vi "PathPlanner_Cmd_FollowHolonomicPathExecute.vi"(5 "PathPlanner_Cmd_FollowHolConfig":T22={"HOLONOMIC_CTRL_PACK_TUNING"={"X PID Tuning"={"Kp"=0.0, "Ki"=0.0, "Kd"=0.0, "MaximumIntegral"=9.9e+30, "MinimumIntegral"=-9.9e+30, "IntegralZone"=9.9e+30}, "Y PID Tuning"={"Kp"=0.0, "Ki"=0.0, "Kd"=0.0, "MaximumIntegral"=9.9e+30, "MinimumIntegral"=-9.9e+30, "IntegralZone"=9.9e+30}, "thetaProfiledPID_CTRL"={"Controller"={"Kp"=0.0, "Ki"=0.0, "Kd"=0.0, "Period"=0.0, "Max_Integral"=1.0, "Min_Integral"=-1.0, "Max_Input"=0.0, "Min_Input"=0.0, "Continuous"=FALSE, "PositionError"=0.0, "VelocityError"=0.0, "PrevError"=0.0, "Total_Integral"=0.0, "PositionTolerance"=0.05, "VelocityTolerance"=9.99e+35, "SetPoint"=0.0, "Kf"=0.0, "Prev_Deriv"=0.0, "Prev_Deriv 2"=0.0, "DerivativeFilter"=FALSE, "Min_Output"=-9.99e+35, "Max_Output"=9.9e+35, "Prev_F_P"=0.0, "Prev_F_P_2"=0.0, "AntiWindupActive"=FALSE, "Measurement"=0.0, "IntegralZone"=9.9e+30}, "Goal"={"Position"=0.0, "Velocity"=0.0}, "Setpoint"={"Position"=0.0, "Velocity"=0.0}, "Constraint"={"MaxVelocity"=0.0, "MaxAcceleration"=0.0}}}, "Max Wheel Speed M/S"=0.0, "Tolerance SI"={"TRANSLATION"={"X"=0.04, "Y"=0.04}, "ROTATION"={"VALUE"=0.034906585039887, "COS"=0.999390827019096, "SIN"=0.034899496702501}}, "Drive Base Radius M"=0.0, "ControlPastEnd_Sec"=3.0, "ReplanningConfig"={"enableInitialReplanning"=FALSE, "enableDynamicReplanning"=FALSE, "dynamicReplanningTotalErrorThreshold"=0.0, "dynamicReplanningErrorSpikeThreshold"=0.0}, "Period_Sec"=0.02, "Trigger Events"=TRUE} {"Tolerance SI"."ROTATION"."SIN" format="%13.4f"; "Tolerance SI"."ROTATION"."COS" format="%13.4f"; "Tolerance SI"."ROTATION"."VALUE" format="%13.4f"; "Tolerance SI"."TRANSLATION"."Y" format="%14.3f"; "Tolerance SI"."TRANSLATION"."X" format="%14.3f"; "HOLONOMIC_CTRL_PACK_TUNING"."thetaProfiledPID_CTRL"."Constraint"."MaxAcceleration" format="%16_6e"; "HOLONOMIC_CTRL_PACK_TUNING"."thetaProfiledPID_CTRL"."Constraint"."MaxVelocity" format="%16_6e"; "HOLONOMIC_CTRL_PACK_TUNING"."thetaProfiledPID_CTRL"."Setpoint"."Velocity" format="%16_6e"; "HOLONOMIC_CTRL_PACK_TUNING"."thetaProfiledPID_CTRL"."Setpoint"."Position" format="%16_6e"; "HOLONOMIC_CTRL_PACK_TUNING"."thetaProfiledPID_CTRL"."Goal"."Velocity" format="%16_6e"; "HOLONOMIC_CTRL_PACK_TUNING"."thetaProfiledPID_CTRL"."Goal"."Position" format="%16_6e"; "HOLONOMIC_CTRL_PACK_TUNING"."thetaProfiledPID_CTRL"."Controller"."IntegralZone" format="%16_6e"; "HOLONOMIC_CTRL_PACK_TUNING"."thetaProfiledPID_CTRL"."Controller"."Measurement" format="%16_6e"; "HOLONOMIC_CTRL_PACK_TUNING"."thetaProfiledPID_CTRL"."Controller"."Prev_F_P_2" format="%16_6e"; "HOLONOMIC_CTRL_PACK_TUNING"."thetaProfiledPID_CTRL"."Controller"."Prev_F_P" format="%16_6e"; "HOLONOMIC_CTRL_PACK_TUNING"."thetaProfiledPID_CTRL"."Controller"."Max_Output" format="%16_6e"; "HOLONOMIC_CTRL_PACK_TUNING"."thetaProfiledPID_CTRL"."Controller"."Min_Output" format="%16_6e"; "HOLONOMIC_CTRL_PACK_TUNING"."thetaProfiledPID_CTRL"."Controller"."Prev_Deriv 2" format="%16_6e"; "HOLONOMIC_CTRL_PACK_TUNING"."thetaProfiledPID_CTRL"."Controller"."Prev_Deriv" format="%16_6e"; "HOLONOMIC_CTRL_PACK_TUNING"."thetaProfiledPID_CTRL"."Controller"."Kf" format="%16_6e"; "HOLONOMIC_CTRL_PACK_TUNING"."thetaProfiledPID_CTRL"."Controller"."SetPoint" format="%16_6e"; "HOLONOMIC_CTRL_PACK_TUNING"."thetaProfiledPID_CTRL"."Controller"."VelocityTolerance" format="%16_6e"; "HOLONOMIC_CTRL_PACK_TUNING"."thetaProfiledPID_CTRL"."Controller"."PositionTolerance" format="%16_6e"; "HOLONOMIC_CTRL_PACK_TUNING"."thetaProfiledPID_CTRL"."Controller"."Total_Integral" format="%16_6e"; "HOLONOMIC_CTRL_PACK_TUNING"."thetaProfiledPID_CTRL"."Controller"."PrevError" format="%16_6e"; "HOLONOMIC_CTRL_PACK_TUNING"."thetaProfiledPID_CTRL"."Controller"."VelocityError" format="%16_6e"; "HOLONOMIC_CTRL_PACK_TUNING"."thetaProfiledPID_CTRL"."Controller"."PositionError" format="%16_6e"; "HOLONOMIC_CTRL_PACK_TUNING"."thetaProfiledPID_CTRL"."Controller"."Min_Input" format="%16_6e"; "HOLONOMIC_CTRL_PACK_TUNING"."thetaProfiledPID_CTRL"."Controller"."Max_Input" format="%16_6e"; "HOLONOMIC_CTRL_PACK_TUNING"."thetaProfiledPID_CTRL"."Controller"."Min_Integral" format="%16_6e"; "HOLONOMIC_CTRL_PACK_TUNING"."thetaProfiledPID_CTRL"."Controller"."Max_Integral" format="%16_6e"; "HOLONOMIC_CTRL_PACK_TUNING"."thetaProfiledPID_CTRL"."Controller"."Period" format="%16_6e"; "HOLONOMIC_CTRL_PACK_TUNING"."thetaProfiledPID_CTRL"."Controller"."Kd" format="%16_6e"; "HOLONOMIC_CTRL_PACK_TUNING"."thetaProfiledPID_CTRL"."Controller"."Ki" format="%16_6e"; "HOLONOMIC_CTRL_PACK_TUNING"."thetaProfiledPID_CTRL"."Controller"."Kp" format="%16_6e"}, 6 "PassthroughTime_SEC":dbl=-1.0, 7 "PathPlannerPath":T2={"Reversed"=FALSE, "RotationTargets"=[], "ConstraintZones"=[], "EventMarkers"=[], "GlobalConstraints"={"MaxVelocityMps;"=0.0, "MaxAccelerationMpsSq;"=0.0, "MaxAngularVelRadPsEc;"=0.0, "MaxAngularAccRadPSecSq"=0.0, "Exists"=FALSE, "Unlimited"=FALSE, "NominalVoltageVolts"=12.0}, "GoalEndState"={"VelocityMPS"=0.0, "Rotation"={"VALUE"=0.0, "COS"=1.0, "SIN"=0.0}}, "AllPoints"=[], "Name"="", "Waypoints"=[], "PointTowardsZones"=[], "IdealStartingState"={"VelocityMPS"=0.0, "Rotation"={"VALUE"=1.0, "COS"=0.0, "SIN"=0.0}}, "IsChoreoPath"=FALSE, "PreventFlipping"=FALSE} {"IdealStartingState"."Rotation"."SIN" format="%13.4f"; "IdealStartingState"."Rotation"."COS" format="%13.4f"; "IdealStartingState"."Rotation"."VALUE" format="%13.4f"; "PointTowardsZones"."TargetPosition"."Y" format="%14.3f"; "PointTowardsZones"."TargetPosition"."X" format="%14.3f"; "PointTowardsZones"."RotationOffset"."SIN" format="%13.4f"; "PointTowardsZones"."RotationOffset"."COS" format="%13.4f"; "PointTowardsZones"."RotationOffset"."VALUE" format="%13.4f"; "Waypoints"."nextControl"."Y" format="%14.3f"; "Waypoints"."nextControl"."X" format="%14.3f"; "Waypoints"."anchor"."Y" format="%14.3f"; "Waypoints"."anchor"."X" format="%14.3f"; "Waypoints"."prevControl"."Y" format="%14.3f"; "Waypoints"."prevControl"."X" format="%14.3f"; "AllPoints"."RotationTarget"."rotation"."SIN" format="%13.4f"; "AllPoints"."RotationTarget"."rotation"."COS" format="%13.4f"; "AllPoints"."RotationTarget"."rotation"."VALUE" format="%13.4f"; "AllPoints"."Position"."Y" format="%14.3f"; "AllPoints"."Position"."X" format="%14.3f"; "GoalEndState"."Rotation"."SIN" format="%13.4f"; "GoalEndState"."Rotation"."COS" format="%13.4f"; "GoalEndState"."Rotation"."VALUE" format="%13.4f"; "RotationTargets"."rotation"."SIN" format="%13.4f"; "RotationTargets"."rotation"."COS" format="%13.4f"; "RotationTargets"."rotation"."VALUE" format="%13.4f"}, 8 "Enabled":bool=TRUE, 9 "Reset":bool, 10 "CurrentChassisSpeeds":T1 {"vOmega" format="%10.3f"; "vY" format="%10.3f"; "vX" format="%10.3f"}, 11 "Current Pose SI":T17={"TRANSLATION"={"X"=0.0, "Y"=0.0}, "ROTATION"={"VALUE"=0.0, "COS"=1.0, "SIN"=0.0}} {"ROTATION"."SIN" format="%13.4f"; "ROTATION"."COS" format="%13.4f"; "ROTATION"."VALUE" format="%13.4f"; "TRANSLATION"."Y" format="%14.3f"; "TRANSLATION"."X" format="%14.3f"}) -> (0 "Position Error M":dbl, 1 "Complete":bool, 2 "At Reference":bool, 3 "calcChassisSpeed":T1 {"vOmega" format="%10.3f"; "vY" format="%10.3f"; "vX" format="%10.3f"}, 4 "outHOLONOMIC_DRV_CTRL":T16={"poseTolerance"={"TRANSLATION"={"X"=0.0, "Y"=0.0}, "ROTATION"={"VALUE"=0.0, "COS"=1.0, "SIN"=0.0}}, "poseError"={"TRANSLATION"={"X"=0.0, "Y"=0.0}, "ROTATION"={"VALUE"=0.0, "COS"=1.0, "SIN"=0.0}}, "Enabled"=TRUE, "PID_xCtrl"={"Kp"=0.0, "Ki"=0.0, "Kd"=0.0, "Period"=0.0, "Max_Integral"=1.0, "Min_Integral"=-1.0, "Max_Input"=0.0, "Min_Input"=0.0, "Continuous"=FALSE, "PositionError"=0.0, "VelocityError"=0.0, "PrevError"=0.0, "Total_Integral"=0.0, "PositionTolerance"=0.05, "VelocityTolerance"=9.99e+35, "SetPoint"=0.0, "Kf"=0.0, "Prev_Deriv"=0.0, "Prev_Deriv 2"=0.0, "DerivativeFilter"=FALSE, "Min_Output"=-9.99e+35, "Max_Output"=9.9e+35, "Prev_F_P"=0.0, "Prev_F_P_2"=0.0, "AntiWindupActive"=FALSE, "Measurement"=0.0, "IntegralZone"=9.9e+30}, "PID_yCtrl"={"Kp"=0.0, "Ki"=0.0, "Kd"=0.0, "Period"=0.0, "Max_Integral"=1.0, "Min_Integral"=-1.0, "Max_Input"=0.0, "Min_Input"=0.0, "Continuous"=FALSE, "PositionError"=0.0, "VelocityError"=0.0, "PrevError"=0.0, "Total_Integral"=0.0, "PositionTolerance"=0.05, "VelocityTolerance"=9.99e+35, "SetPoint"=0.0, "Kf"=0.0, "Prev_Deriv"=0.0, "Prev_Deriv 2"=0.0, "DerivativeFilter"=FALSE, "Min_Output"=-9.99e+35, "Max_Output"=9.9e+35, "Prev_F_P"=0.0, "Prev_F_P_2"=0.0, "AntiWindupActive"=FALSE, "Measurement"=0.0, "IntegralZone"=9.9e+30}, "PROF_PID_thetaCtrl"={"Controller"={"Kp"=0.0, "Ki"=0.0, "Kd"=0.0, "Period"=0.0, "Max_Integral"=1.0, "Min_Integral"=-1.0, "Max_Input"=0.0, "Min_Input"=0.0, "Continuous"=FALSE, "PositionError"=0.0, "VelocityError"=0.0, "PrevError"=0.0, "Total_Integral"=0.0, "PositionTolerance"=0.05, "VelocityTolerance"=9.99e+35, "SetPoint"=0.0, "Kf"=0.0, "Prev_Deriv"=0.0, "Prev_Deriv 2"=0.0, "DerivativeFilter"=FALSE, "Min_Output"=-9.99e+35, "Max_Output"=9.9e+35, "Prev_F_P"=0.0, "Prev_F_P_2"=0.0, "AntiWindupActive"=FALSE, "Measurement"=0.0, "IntegralZone"=9.9e+30}, "Goal"={"Position"=0.0, "Velocity"=0.0}, "Setpoint"={"Position"=0.0, "Velocity"=0.0}, "Constraint"={"MaxVelocity"=0.0, "MaxAcceleration"=0.0}}, "RotationError"={"VALUE"=0.0, "COS"=1.0, "SIN"=0.0}, "FirstRun"=TRUE} {"RotationError"."SIN" format="%13.4f"; "RotationError"."COS" format="%13.4f"; "RotationError"."VALUE" format="%13.4f"; "PROF_PID_thetaCtrl"."Constraint"."MaxAcceleration" format="%16_6e"; "PROF_PID_thetaCtrl"."Constraint"."MaxVelocity" format="%16_6e"; "PROF_PID_thetaCtrl"."Setpoint"."Velocity" format="%16_6e"; "PROF_PID_thetaCtrl"."Setpoint"."Position" format="%16_6e"; "PROF_PID_thetaCtrl"."Goal"."Velocity" format="%16_6e"; "PROF_PID_thetaCtrl"."Goal"."Position" format="%16_6e"; "PROF_PID_thetaCtrl"."Controller"."IntegralZone" format="%16_6e"; "PROF_PID_thetaCtrl"."Controller"."Measurement" format="%16_6e"; "PROF_PID_thetaCtrl"."Controller"."Prev_F_P_2" format="%16_6e"; "PROF_PID_thetaCtrl"."Controller"."Prev_F_P" format="%16_6e"; "PROF_PID_thetaCtrl"."Controller"."Max_Output" format="%16_6e"; "PROF_PID_thetaCtrl"."Controller"."Min_Output" format="%16_6e"; "PROF_PID_thetaCtrl"."Controller"."Prev_Deriv 2" format="%16_6e"; "PROF_PID_thetaCtrl"."Controller"."Prev_Deriv" format="%16_6e"; "PROF_PID_thetaCtrl"."Controller"."Kf" format="%16_6e"; "PROF_PID_thetaCtrl"."Controller"."SetPoint" format="%16_6e"; "PROF_PID_thetaCtrl"."Controller"."VelocityTolerance" format="%16_6e"; "PROF_PID_thetaCtrl"."Controller"."PositionTolerance" format="%16_6e"; "PROF_PID_thetaCtrl"."Controller"."Total_Integral" format="%16_6e"; "PROF_PID_thetaCtrl"."Controller"."PrevError" format="%16_6e"; "PROF_PID_thetaCtrl"."Controller"."VelocityError" format="%16_6e"; "PROF_PID_thetaCtrl"."Controller"."PositionError" format="%16_6e"; "PROF_PID_thetaCtrl"."Controller"."Min_Input" format="%16_6e"; "PROF_PID_thetaCtrl"."Controller"."Max_Input" format="%16_6e"; "PROF_PID_thetaCtrl"."Controller"."Min_Integral" format="%16_6e"; "PROF_PID_thetaCtrl"."Controller"."Max_Integral" format="%16_6e"; "PROF_PID_thetaCtrl"."Controller"."Period" format="%16_6e"; "PROF_PID_thetaCtrl"."Controller"."Kd" format="%16_6e"; "PROF_PID_thetaCtrl"."Controller"."Ki" format="%16_6e"; "PROF_PID_thetaCtrl"."Controller"."Kp" format="%16_6e"; "PID_yCtrl"."IntegralZone" format="%16_6e"; "PID_yCtrl"."Measurement" format="%16_6e"; "PID_yCtrl"."Prev_F_P_2" format="%16_6e"; "PID_yCtrl"."Prev_F_P" format="%16_6e"; "PID_yCtrl"."Max_Output" format="%16_6e"; "PID_yCtrl"."Min_Output" format="%16_6e"; "PID_yCtrl"."Prev_Deriv 2" format="%16_6e"; "PID_yCtrl"."Prev_Deriv" format="%16_6e"; "PID_yCtrl"."Kf" format="%16_6e"; "PID_yCtrl"."SetPoint" format="%16_6e"; "PID_yCtrl"."VelocityTolerance" format="%16_6e"; "PID_yCtrl"."PositionTolerance" format="%16_6e"; "PID_yCtrl"."Total_Integral" format="%16_6e"; "PID_yCtrl"."PrevError" format="%16_6e"; "PID_yCtrl"."VelocityError" format="%16_6e"; "PID_yCtrl"."PositionError" format="%16_6e"; "PID_yCtrl"."Min_Input" format="%16_6e"; "PID_yCtrl"."Max_Input" format="%16_6e"; "PID_yCtrl"."Min_Integral" format="%16_6e"; "PID_yCtrl"."Max_Integral" format="%16_6e"; "PID_yCtrl"."Period" format="%16_6e"; "PID_yCtrl"."Kd" format="%16_6e"; "PID_yCtrl"."Ki" format="%16_6e"; "PID_yCtrl"."Kp" format="%16_6e"; "PID_xCtrl"."IntegralZone" format="%16_6e"; "PID_xCtrl"."Measurement" format="%16_6e"; "PID_xCtrl"."Prev_F_P_2" format="%16_6e"; "PID_xCtrl"."Prev_F_P" format="%16_6e"; "PID_xCtrl"."Max_Output" format="%16_6e"; "PID_xCtrl"."Min_Output" format="%16_6e"; "PID_xCtrl"."Prev_Deriv 2" format="%16_6e"; "PID_xCtrl"."Prev_Deriv" format="%16_6e"; "PID_xCtrl"."Kf" format="%16_6e"; "PID_xCtrl"."SetPoint" format="%16_6e"; "PID_xCtrl"."VelocityTolerance" format="%16_6e"; "PID_xCtrl"."PositionTolerance" format="%16_6e"; "PID_xCtrl"."Total_Integral" format="%16_6e"; "PID_xCtrl"."PrevError" format="%16_6e"; "PID_xCtrl"."VelocityError" format="%16_6e"; "PID_xCtrl"."PositionError" format="%16_6e"; "PID_xCtrl"."Min_Input" format="%16_6e"; "PID_xCtrl"."Max_Input" format="%16_6e"; "PID_xCtrl"."Min_Integral" format="%16_6e"; "PID_xCtrl"."Max_Integral" format="%16_6e"; "PID_xCtrl"."Period" format="%16_6e"; "PID_xCtrl"."Kd" format="%16_6e"; "PID_xCtrl"."Ki" format="%16_6e"; "PID_xCtrl"."Kp" format="%16_6e"; "poseError"."ROTATION"."SIN" format="%13.4f"; "poseError"."ROTATION"."COS" format="%13.4f"; "poseError"."ROTATION"."VALUE" format="%13.4f"; "poseError"."TRANSLATION"."Y" format="%14.3f"; "poseError"."TRANSLATION"."X" format="%14.3f"; "poseTolerance"."ROTATION"."SIN" format="%13.4f"; "poseTolerance"."ROTATION"."COS" format="%13.4f"; "poseTolerance"."ROTATION"."VALUE" format="%13.4f"; "poseTolerance"."TRANSLATION"."Y" format="%14.3f"; "poseTolerance"."TRANSLATION"."X" format="%14.3f"})   [LabVIEW 2019, in "PathPlanner24.lvlib"]
doc: "DOCUMENTATION IS NOT COMPLETE.\n \nCalculates the next output of the path following controller for holonomic drive robots. This wraps a Holonomic Drive Control function with the particulars needed to follow a PathPlanner trajectory.\n\nInputs:\n - PathPlanner_Holonomic_Ctrl_Pack_Tuning - cluster - The tuning paraameters for the holonomic drive controller. These are static. They should not be changed after the first call to this function.\n - CurrentPoseSi - pose2d - The current pose calculated by odometry or pose estimation. The pose can be absolute or relative depending on what type of trajectory is being followed.\n - PathPlannerState - cluster - The path palnner trajectory state containing the desired position and velocities of the robot.\n - Reset - boolean - When TRUE the holonomic drive controller is reset. This should be set to TRUE for the first execution of a trajectory.\n - Enabled - boolean - When TRUE, closed loop control is enabled. (Optional. Default: TRUE)\n - Period - double - The loop period in seconds for this controller. (Optional. Default: 0.020)\n\nOutputs:\n - CalcChassisSpeed - cluster - The desired chassis speed in SI units.\n - AtReference - boolean - TRUE if the robots position is within the defined tolerance.\n - PositionError - pose2d - Position error in SI units. How far the robot is away from the desired trajectory position.\n - out_Holonomic_Drive_Ctrl - THe current holonomic drive controller data cluster. This is mainly for diagnostic purposes."
uses:
  PathPlanner24.lvlib
  <vilib>/Rock Robotics/WPI/ThirdParty/JAS_Junk/TrajLib/TypeDef/TRANSLATION2D.ctl
  <vilib>/Rock Robotics/WPI/ThirdParty/JAS_Junk/TrajLib/Trajectory_Library.lvlib
  <vilib>/Rock Robotics/WPI/ThirdParty/JAS_Junk/TrajLib/TypeDef/ROTATION2D.ctl
  <vilib>/Rock Robotics/WPI/ThirdParty/JAS_Junk/TrajLib/TypeDef/POSE2D.ctl
  <vilib>/Rock Robotics/WPI/ThirdParty/JAS_Junk/TrajLib/TypeDef/PID_TUNING.ctl
  <vilib>/Rock Robotics/WPI/ThirdParty/JAS_Junk/TrajLib/TypeDef/PID_CONTROLLER.ctl
  <vilib>/Rock Robotics/WPI/ThirdParty/JAS_Junk/TrajLib/TypeDef/TRAPEZOID_PROFILE_STATE.ctl
  <vilib>/Rock Robotics/WPI/ThirdParty/JAS_Junk/TrajLib/TypeDef/TRAPEZOID_PROFILE_CONSTRAINT.ctl
  <vilib>/Rock Robotics/WPI/ThirdParty/JAS_Junk/TrajLib/TypeDef/PROFILED_PID_CONTROLLER.ctl
  <vilib>/Rock Robotics/WPI/ThirdParty/JAS_Junk/TrajLib/TypeDef/HOLONOMIC_PACK_TUNING.ctl
  <vilib>/Rock Robotics/WPI/ThirdParty/JAS_Junk/TrajLib/TypeDef/HOLONOMIC_DRV_CTRL.ctl
  <vilib>/Rock Robotics/WPI/ThirdParty/JAS_Junk/TrajLib/TypeDef/CHASSIS_SPEEDS.ctl
  TypeDef/PathPlannerRotationTarget.ctl
  TypeDef/PathPlannerPathConstraints.ctl
  TypeDef/PathPlannerConstraintsZone.ctl
  ENum/PathPlanner_CommandUtilType_ENUM.ctl
  TypeDef/PathPlannerCommandUtil.ctl
  TypeDef/PathPlannerEventMarker.ctl
  TypeDef/PathPlannerGoalEndState.ctl
  TypeDef/PathPlannerPathPoint.ctl
  TypeDef/PathPlannerPath.ctl
  TypeDef/PathPlannerCmdFollowHolConfig.ctl
  TypeDef/PathPlannerReplanningConfig.ctl
  TypeDef/PathPlannerWaypoint.ctl
  TypeDef/PathPlannerPointTowardsZone.ctl
  TypeDef/PathPlannerIdealStartingState.ctl
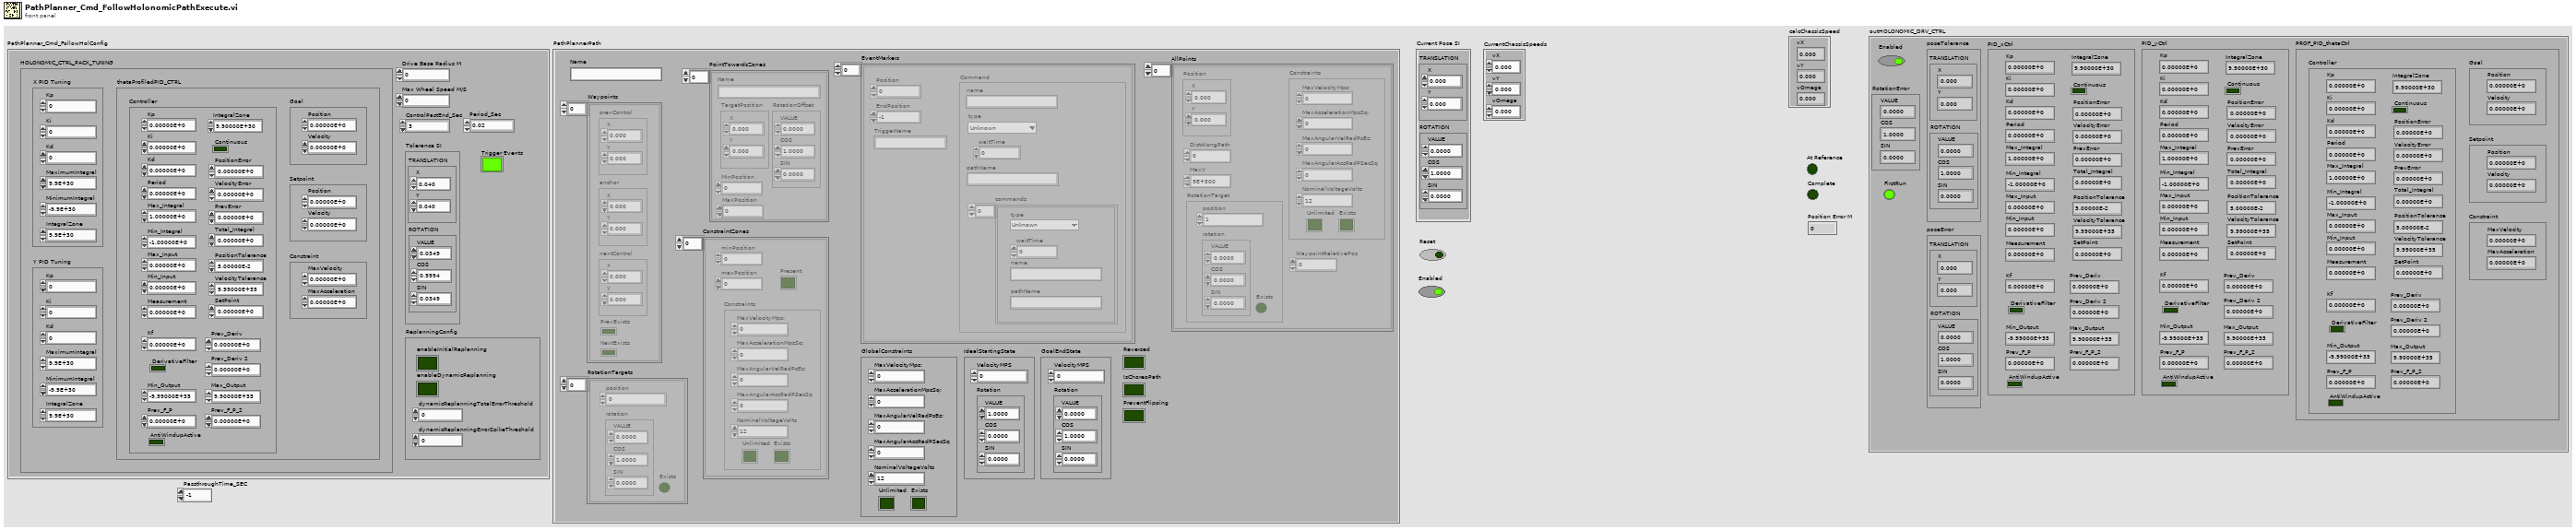
[diagram p1: front panel]
types:
  T1 = typedef "Trajectory_Library.lvlib/CHASSIS_SPEEDS.ctl" = cluster{"vX":dbl, "vY":dbl, "vOmega":dbl}
  T2 = typedef "PathPlanner24.lvlib/PathPlannerPath.ctl" = cluster{"Reversed":bool, "RotationTargets":T3[], "ConstraintZones":T5[], "EventMarkers":T7[], "GlobalConstraints":T6, "GoalEndState":T10, "AllPoints":T11[], "Name":string, "Waypoints":T13[], "PointTowardsZones":T14[], "IdealStartingState":T15, "IsChoreoPath":bool, "PreventFlipping":bool}
  T3 = typedef "PathPlanner24.lvlib/PathPlannerRotationTarget.ctl" = cluster{"position":dbl, "rotation":T4, "Exists":bool}
  T4 = typedef "Trajectory_Library.lvlib/ROTATION2D.ctl" = cluster{"VALUE":dbl, "COS":dbl, "SIN":dbl}
  T5 = typedef "PathPlanner24.lvlib/PathPlannerConstraintsZone.ctl" = cluster{"minPosition":dbl, "maxPosition":dbl, "Constraints":T6, "Present":bool}
  T6 = typedef "PathPlanner24.lvlib/PathPlannerPathConstraints.ctl" = cluster{"MaxVelocityMps;":dbl, "MaxAccelerationMpsSq;":dbl, "MaxAngularVelRadPsEc;":dbl, "MaxAngularAccRadPSecSq":dbl, "Exists":bool, "Unlimited":bool, "NominalVoltageVolts":dbl}
  T7 = typedef "PathPlanner24.lvlib/PathPlannerEventMarker.ctl" = cluster{"Position":dbl, "Command":T8, "TriggerName":string, "EndPosition":dbl}
  T8 = typedef "PathPlanner24.lvlib/PathPlannerCommandUtil.ctl" = cluster{"waitTime":dbl, "name":string, "pathName":string, "commands":cluster{"type":T9, "waitTime":dbl, "name":string, "pathName":string}[], "type":T9}
  T9 = typedef "PathPlanner24.lvlib/PathPlanner_CommandUtilType_ENUM.ctl" = enum16{"Unknown", "Wait", "Named", "Path", "Sequential", "Parallel", "Race", "Deadline"}
  T10 = typedef "PathPlanner24.lvlib/PathPlannerGoalEndState.ctl" = cluster{"VelocityMPS":dbl, "Rotation":T4}
  T11 = typedef "PathPlanner24.lvlib/PathPlannerPathPoint.ctl" = cluster{"Position":T12, "DistAlongPath":dbl, "MaxV":dbl, "Constraints":T6, "RotationTarget":T3, "WaypointRelativePos":dbl}
  T12 = typedef "Trajectory_Library.lvlib/TRANSLATION2D.ctl" = cluster{"X":dbl, "Y":dbl}
  T13 = typedef "PathPlanner24.lvlib/PathPlannerWaypoint.ctl" = cluster{"prevControl":T12, "anchor":T12, "nextControl":T12, "PrevExists":bool, "NextExists":bool}
  T14 = typedef "PathPlanner24.lvlib/PathPlannerPointTowardsZone.ctl" = cluster{"RotationOffset":T4, "Name":string, "TargetPosition":T12, "MinPosition":dbl, "MaxPosition":dbl}
  T15 = typedef "PathPlanner24.lvlib/PathPlannerIdealStartingState.ctl" = cluster{"VelocityMPS":dbl, "Rotation":T4}
  T16 = typedef "Trajectory_Library.lvlib/HOLONOMIC_DRV_CTRL.ctl" = cluster{"poseTolerance":T17, "poseError":T17, "Enabled":bool, "PID_xCtrl":T18, "PID_yCtrl":T18, "PROF_PID_thetaCtrl":T19, "RotationError":T4, "FirstRun":bool}
  T17 = typedef "Trajectory_Library.lvlib/POSE2D.ctl" = cluster{"TRANSLATION":T12, "ROTATION":T4}
  T18 = typedef "Trajectory_Library.lvlib/PID_CONTROLLER.ctl" = cluster{"Kp":dbl, "Ki":dbl, "Kd":dbl, "Period":dbl, "Max_Integral":dbl, "Min_Integral":dbl, "Max_Input":dbl, "Min_Input":dbl, "Continuous":bool, "PositionError":dbl, "VelocityError":dbl, "PrevError":dbl, "Total_Integral":dbl, "PositionTolerance":dbl, "VelocityTolerance":dbl, "SetPoint":dbl, "Kf":dbl, "Prev_Deriv":dbl, "Prev_Deriv 2":dbl, "DerivativeFilter":bool, "Min_Output":dbl, "Max_Output":dbl, "Prev_F_P":dbl, "Prev_F_P_2":dbl, "AntiWindupActive":bool, "Measurement":dbl, "IntegralZone":dbl}
  T19 = typedef "Trajectory_Library.lvlib/PROFILED_PID_CONTROLLER.ctl" = cluster{"Controller":T18, "Goal":T20, "Setpoint":T20, "Constraint":T21}
  T20 = typedef "Trajectory_Library.lvlib/TRAPEZOID_PROFILE_STATE.ctl" = cluster{"Position":dbl, "Velocity":dbl}
  T21 = typedef "Trajectory_Library.lvlib/TRAPEZOID_PROFILE_CONSTRAINT.ctl" = cluster{"MaxVelocity":dbl, "MaxAcceleration":dbl}
  T22 = typedef "PathPlanner24.lvlib/PathPlannerCmdFollowHolConfig.ctl" = cluster{"HOLONOMIC_CTRL_PACK_TUNING":T23, "Max Wheel Speed M/S":dbl, "Tolerance SI":T17, "Drive Base Radius M":dbl, "ControlPastEnd_Sec":dbl, "ReplanningConfig":T25, "Period_Sec":dbl, "Trigger Events":bool}
  T23 = typedef "Trajectory_Library.lvlib/HOLONOMIC_PACK_TUNING.ctl" = cluster{"X PID Tuning":T24, "Y PID Tuning":T24, "thetaProfiledPID_CTRL":T19}
  T24 = typedef "Trajectory_Library.lvlib/PID_TUNING.ctl" = cluster{"Kp":dbl, "Ki":dbl, "Kd":dbl, "MaximumIntegral":dbl, "MinimumIntegral":dbl, "IntegralZone":dbl}
  T25 = typedef "PathPlanner24.lvlib/PathPlannerReplanningConfig.ctl" = cluster{"enableInitialReplanning":bool, "enableDynamicReplanning":bool, "dynamicReplanningTotalErrorThreshold":dbl, "dynamicReplanningErrorSpikeThreshold":dbl}
  T26 = typedef "PathPlanner24.lvlib/PathPlannerCtrlHolConfig.ctl" = cluster{"HOLONOMIC_CTRL_PACK_TUNING":T23, "Max Wheel Speed M/S":dbl, "Tolerance SI":T17, "Drive Base Radius M":dbl}
  T27 = cluster{"Traj Time Plus Extra\nElapsed":bool, "Traj Time Elapsed":bool}
  T28 = typedef "PathPlanner24.lvlib/PathPlannerTrajectoryState24.ctl" = cluster{"TimeSeconds":dbl, "VelocityMPS":dbl, "AccerationMpsSq":dbl, "HeadingAngularVelRadPerSec":dbl, "PositionMeters":T12, "Heading":T4, "TargetHolonomicRotation":T4, "CurvatureRadPerMeter":dbl, "PathPlannerConstraints":T6, "DeltaPos":dbl}
  T29 = typedef "PathPlanner24.lvlib/PathPlannerTrajectoryEvents.ctl" = cluster{"EventCommands":T30[]}
  T30 = typedef "PathPlanner24.lvlib/PathPlannerTrajectoryEvent.ctl" = cluster{"TimeStampSec":dbl, "CommandUtil":T8}
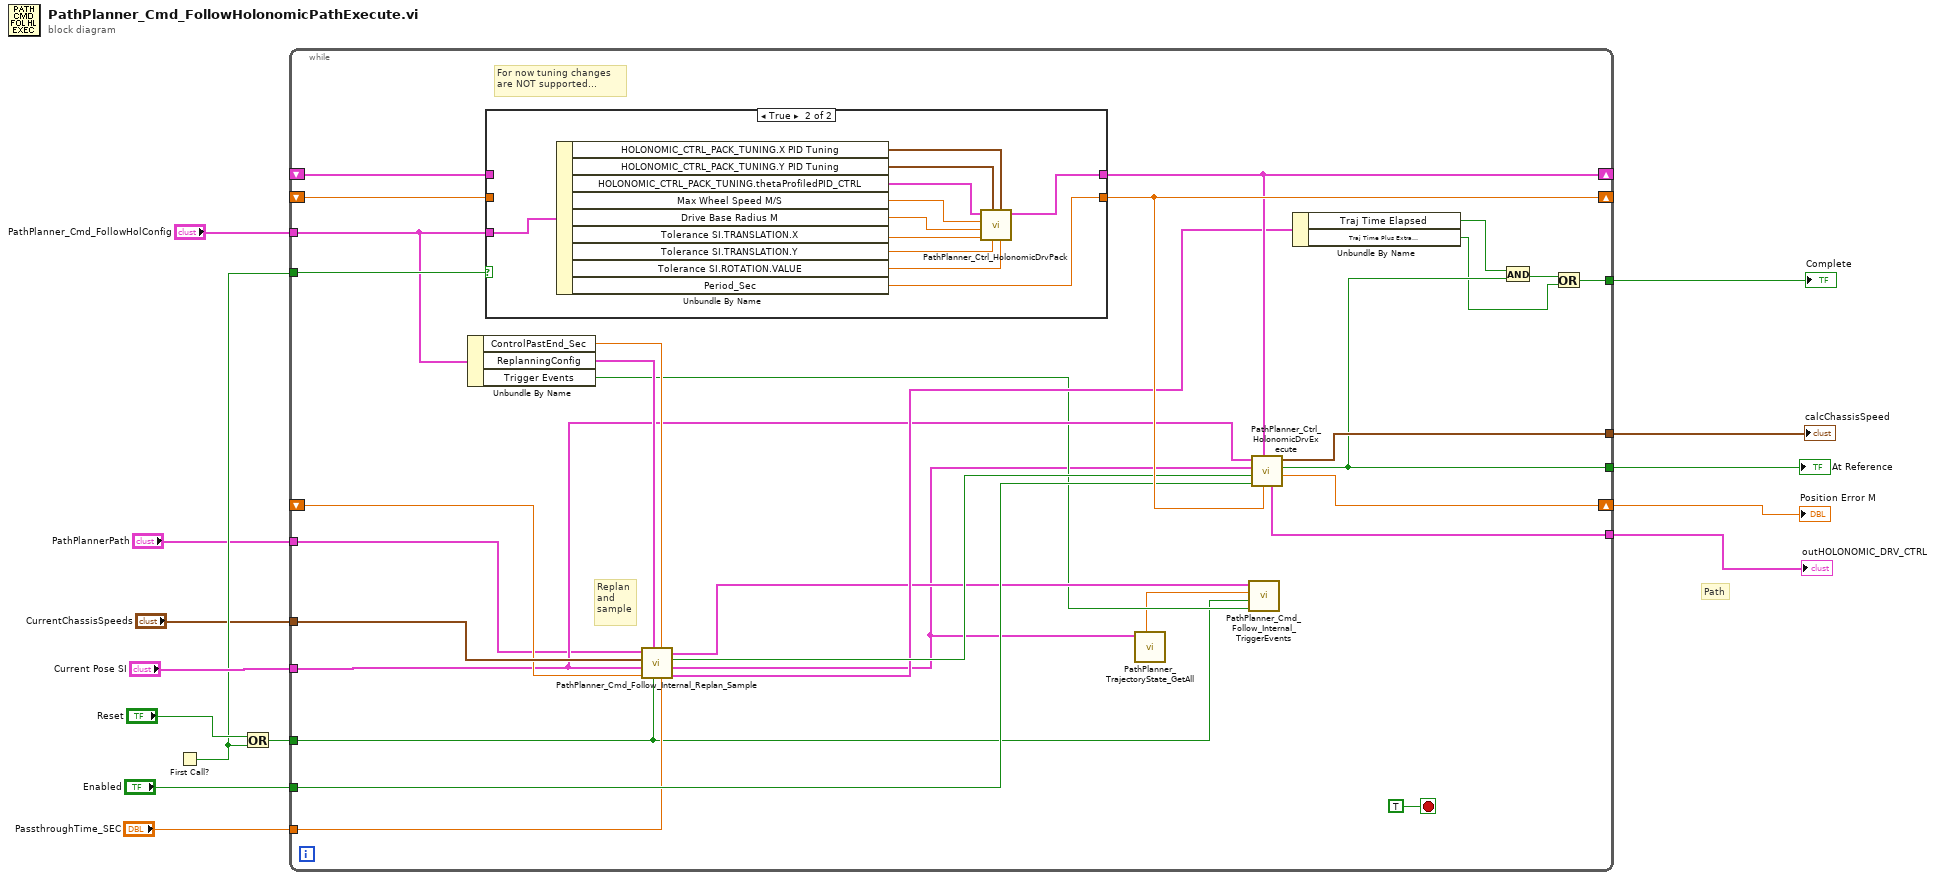
[diagram p0: block diagram]
diagram:
  # "Path"
  n1 = First Call?() -> (First Call?: T/F=w7:bool)
  n2 = Or(x="Reset", y=w7) -> (x .or. y?=w10:bool)
  n3 = while {
    tunnel: "PathPlanner_Cmd_FollowHolConfig" -> [w30]
    tunnel: "Current Pose SI" -> [w20]
    tunnel: [w44] -> w9
    tunnel: w7 -> [w43]
    shift-right: [w40] -> _
    shift-left: _ -> [w39]
    shift-right: [w41] -> _
    shift-left: _ -> [w38]
    tunnel: "Enabled" -> [w37]
    tunnel: [w28] -> w8
    tunnel: "CurrentChassisSpeeds" -> [w33]
    tunnel: "PassthroughTime_SEC" -> [w32]
    tunnel: [w35] -> w4
    shift-right: [w36] -> w5
    shift-left: _ -> [w31]
    tunnel: w10 -> [w17]
    tunnel: "PathPlannerPath" -> [w19]
    tunnel: [w26] -> w1
    stop <- TRUE stop-if-true
    # "Replan\nand \nsample"
    # "For now tuning changes\nare NOT supported..."
    n4 = Unbundle By Name(w30) -> ("ControlPastEnd_Sec"=w22:dbl, "ReplanningConfig"=w29:T25, "Trigger Events"=w18:bool)
    n5 = case shown="True" w43 {
      tunnel: [w46 w50] -> w40
      tunnel: w30 -> [_ w49]
      tunnel: [w45 w48] -> w41
      tunnel: w39 -> [w46 _]
      tunnel: w38 -> [w45 _]
      frame False {
      }
      frame True {
        n6 = Unbundle By Name(w49) -> ("HOLONOMIC_CTRL_PACK_TUNING.X PID Tuning"=w57:T24, "HOLONOMIC_CTRL_PACK_TUNING.Y PID Tuning"=w56:T24, "HOLONOMIC_CTRL_PACK_TUNING.thetaProfiledPID_CTRL"=w55:T19, "Max Wheel Speed M/S"=w54:dbl, "Drive Base Radius M"=w53:dbl, "Tolerance SI.TRANSLATION.X"=w47:dbl, "Tolerance SI.TRANSLATION.Y"=w52:dbl, "Tolerance SI.ROTATION.VALUE"=w51:dbl, "Period_Sec"=w48:dbl)
        n7 = call "PathPlanner_Ctrl_HolonomicDrvPack.vi"("Rotation Tolerance DEG"=w51, "X PID Tuning"=w57, "Y Tolerance M"=w52, "Y PID Tuning"=w56, "X Tolerance M"=w47, "Drive Base Radius M"=w53, "Max Wheel Speed M/S"=w54, "thetaProfiledPID_CTRL"=w55) -> ("PathPlanner_Ctrl_HolDrvConfig"=w50:T26)  [unwired: 3 in]
      }
    }
    n8 = call "PathPlanner_Cmd_Follow_Internal_Replan_Sample.vi"("PassthroughTime_SEC"=w32, "Extra Time Sec"=w22, "Reset In"=w17, "ReplanningConfig"=w29, "Position Error M"=w31, "Current Pose SI"=w20, "CurrentChassisSpeeds"=w33, "RePlannedPath in"=w19) -> ("Traj End Status"=w25:T27, "Trajectory State"=w15:T28, "Reset Controller"=w34:bool, "PathPlannerTrajectoryEvents"=w21:T29)
    n9 = call "PathPlanner_TrajectoryState_GetAll.vi"("PathPlannerState"=w15) -> ("TimeSeconds"=w16:dbl)  [unwired: 1 in, 9 out]
    n10 = call "PathPlanner_Cmd_Follow_Internal_TriggerEvents.vi"("TrigerEvents"=w18, "Reset"=w17, "TrajectoryTimeStampSecs"=w16, "PathPlannerTrajectoryEvents"=w21) -> ()  [unwired: 8 in]
    n11 = call "PathPlanner_Ctrl_HolonomicDrvExecute.vi"("Period"=w41, "PathPlanner_Ctrl_HolDrvConfig"=w40, "Enabled"=w37, "Reset"=w34, "PathPlannerState"=w15, "Current Pose SI"=w20) -> ("Position Error M"=w36:dbl, "At Reference"=w28:bool, "calcChassisSpeed"=w44:T1, "outHOLONOMIC_DRV_CTRL"=w35:T16)  [unwired: 2 in]
    n12 = Unbundle By Name(w25) -> ("Traj Time Elapsed"=w24:bool, "Traj Time Plus Extra\nElapsed"=w23:bool)
    n13 = And(x=w24, y=w28) -> (x .and. y?=w27:bool)
    n14 = Or(x=w27, y=w23) -> (x .or. y?=w26:bool)
  }
  "At Reference" <- w8
  "Position Error M" <- w5
  "outHOLONOMIC_DRV_CTRL" <- w4
  "calcChassisSpeed" <- w9
  "Complete" <- w1
